vi "Read record from DB.vi"(8 "error in (no error)":errorcluster, 10 "Record":T1, 11 "Elevator Controller Actor in":refnum<class "Elevator Controller Actor.lvclass">) -> (0 "error out":errorcluster, 3 "Elevator Controller Actor out":refnum<class "Elevator Controller Actor.lvclass">)   [LabVIEW 2022 SP3, in "Elevator Controller Actor.lvlib" / "Elevator Controller Actor.lvclass"]
uses:
  Elevator Controller Actor.lvclass
  Elevator Controller Actor.lvclass/Elevator Controller Actor.ctl
  Configuration Database Actor/Configuration Database Actor/Record -Cluster.ctl
  Configuration Database Actor/Configuration Database Actor/Configuration Database Actor.lvclass
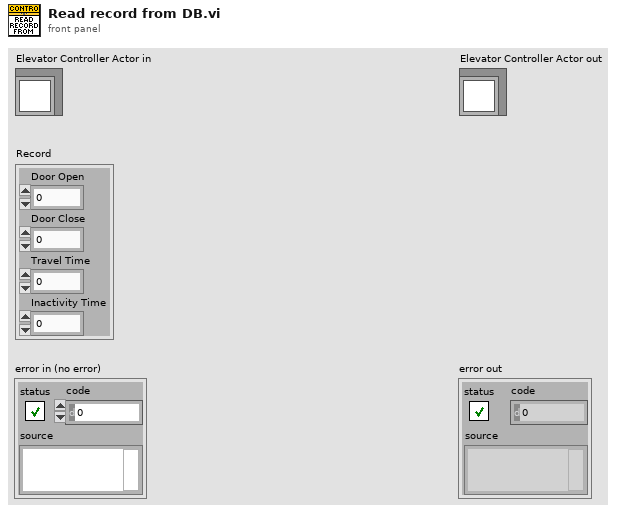
[diagram p1: front panel]
types:
  T1 = typedef "Configuration Database Actor.lvlib/Configuration Database Actor.lvclass/Record -Cluster.ctl" = cluster{"Door Open":dbl, "Door Close":dbl, "Travel Time":dbl, "Inactivity Time":dbl}
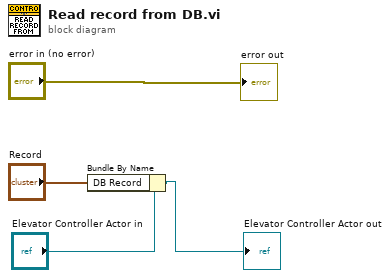
[diagram p0: block diagram]
diagram:
  n1 = Bundle By Name(cluster="Elevator Controller Actor in", "DB Record"="Record") -> (→"Elevator Controller Actor out":refnum<class "Elevator Controller Actor.lvclass">)
  "error out" <- "error in (no error)"
